vi "生产data格式.vi"(11 "data格式选项":T6) -> (3 "表头格式":T1)   [LabVIEW 2017]
panel:
  # "1: 不允许含有中杆"
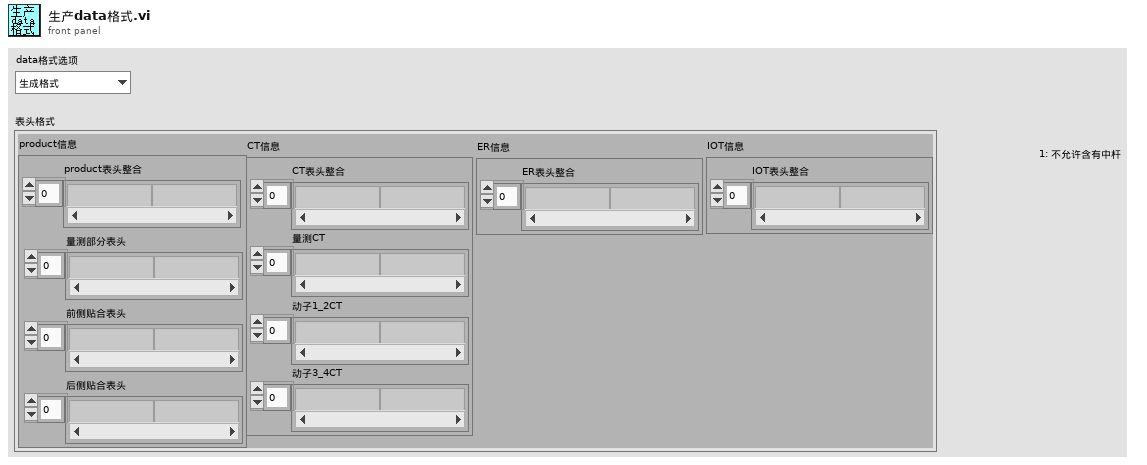
[diagram p1: front panel]
types:
  T1 = typedef "表头集合.ctl" = cluster{"product信息":T2, "CT信息":T3, "ER信息":T4, "IOT信息":T5}
  T2 = typedef "product信息.ctl" = cluster{"product表头整合":string[], "量测部分表头":string[], "前侧贴合表头":string[], "后侧贴合表头":string[]}
  T3 = typedef "CT信息.ctl" = cluster{"CT表头整合":string[], "量测CT":string[], "动子1_2CT":string[], "动子3_4CT":string[]}
  T4 = typedef "ER信息.ctl" = cluster{"ER表头整合":string[]}
  T5 = typedef "IOT信息.ctl" = cluster{"IOT表头整合":string[]}
  T6 = typedef "data格式选项.ctl" = enum16{"生成格式", "加载格式"}
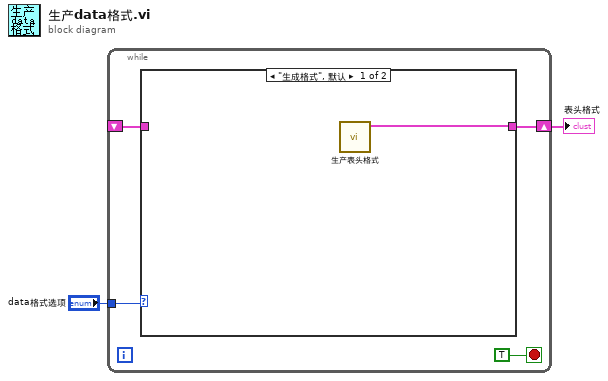
[diagram p0: block diagram]
diagram:
  n1 = while {
    tunnel: "data格式选项" -> [w5]
    shift-right: [w4] -> w1
    shift-left: _ -> [w3]
    stop <- TRUE stop-if-true
    n2 = case shown="\"生成格式\", 默认" w5 {
      tunnel: [w7 w8] -> w4
      tunnel: w3 -> [_ w8]
      frame "生成格式", Default {
        n3 = call "生产表头格式.vi"() -> ("表头格式"=w7:T1)  [unwired: 11 in]
      }
      frame "加载格式" {
      }
    }
  }
  "表头格式" <- w1
